vi "ContactsDC.vi"() -> ()   [LabVIEW 2017]
uses:
  <vilib>/Utility/file.llb/Write To Spreadsheet File (DBL).vi
panel:
  in  "Test first # contacts (#<16)":i8=15
  out "Resistance":dbl
  out "Array":bool[][](array[boolean])
  in  "GPIB Address":string="12"
  out "String":string
  in  "Start testing the contacts":bool
  out "Output Current (A)":dbl
  out "Output Voltage (V)":dbl
  out "Compliance limit (V)":dbl
  out "Current Range":u16(ring) items=["100 nA", "1 uA", "10 uA", "100 uA", "1 mA", "10 mA", "100 mA", "1 A"]
  out "Voltage Range":u16(ring) items=["200 mV", "2 V", "20 V", "200 V"]
  out "Current (sourse)":dbl
  out "Voltage (sourse)":dbl
  out "ComplianceIndicator":bool
  out "Compliance limit (A)":dbl
  out "Source Function":u16(ring)=1 items=["Current Source", "Voltage Source"]
  out "Sence Mode":u16(ring) items=["2-wire", "4-wire"]
  in  "ON/OFF channel":bool
  out "ON/OFF indicator":bool
  in  "error in (no error)":errorcluster
  out "error out":errorcluster
  # "Channel\nB"
  # "Before start testing contacts make sure that voltage 1 mV is set on channel B,\nchannel is ON, and compliance is 1 uA (1E-6 A) or smaller."
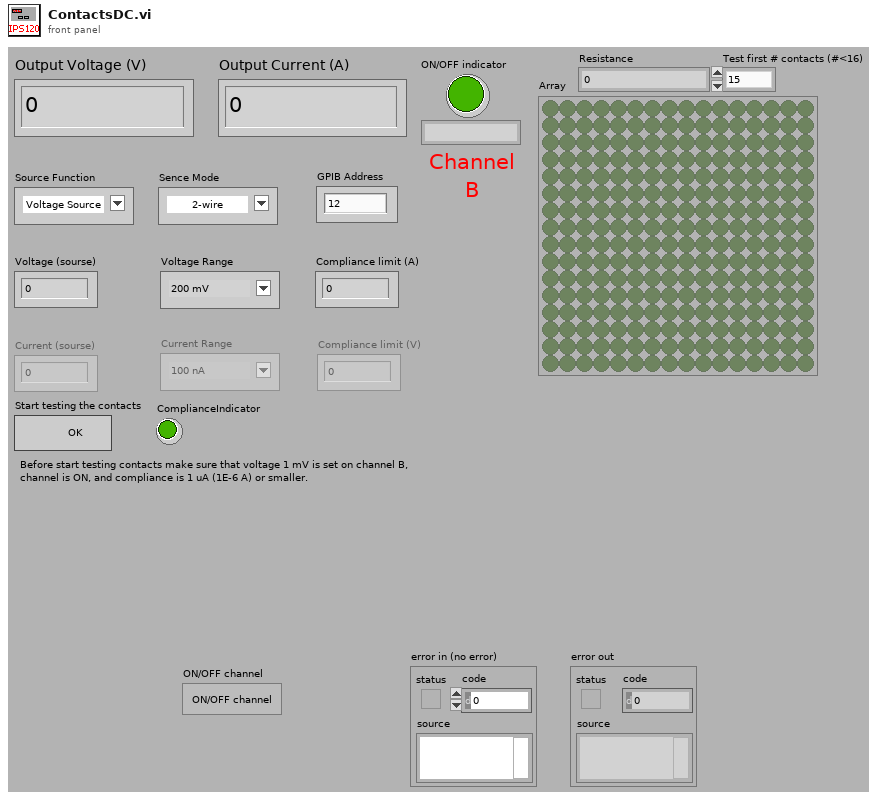
[diagram p1: front panel]
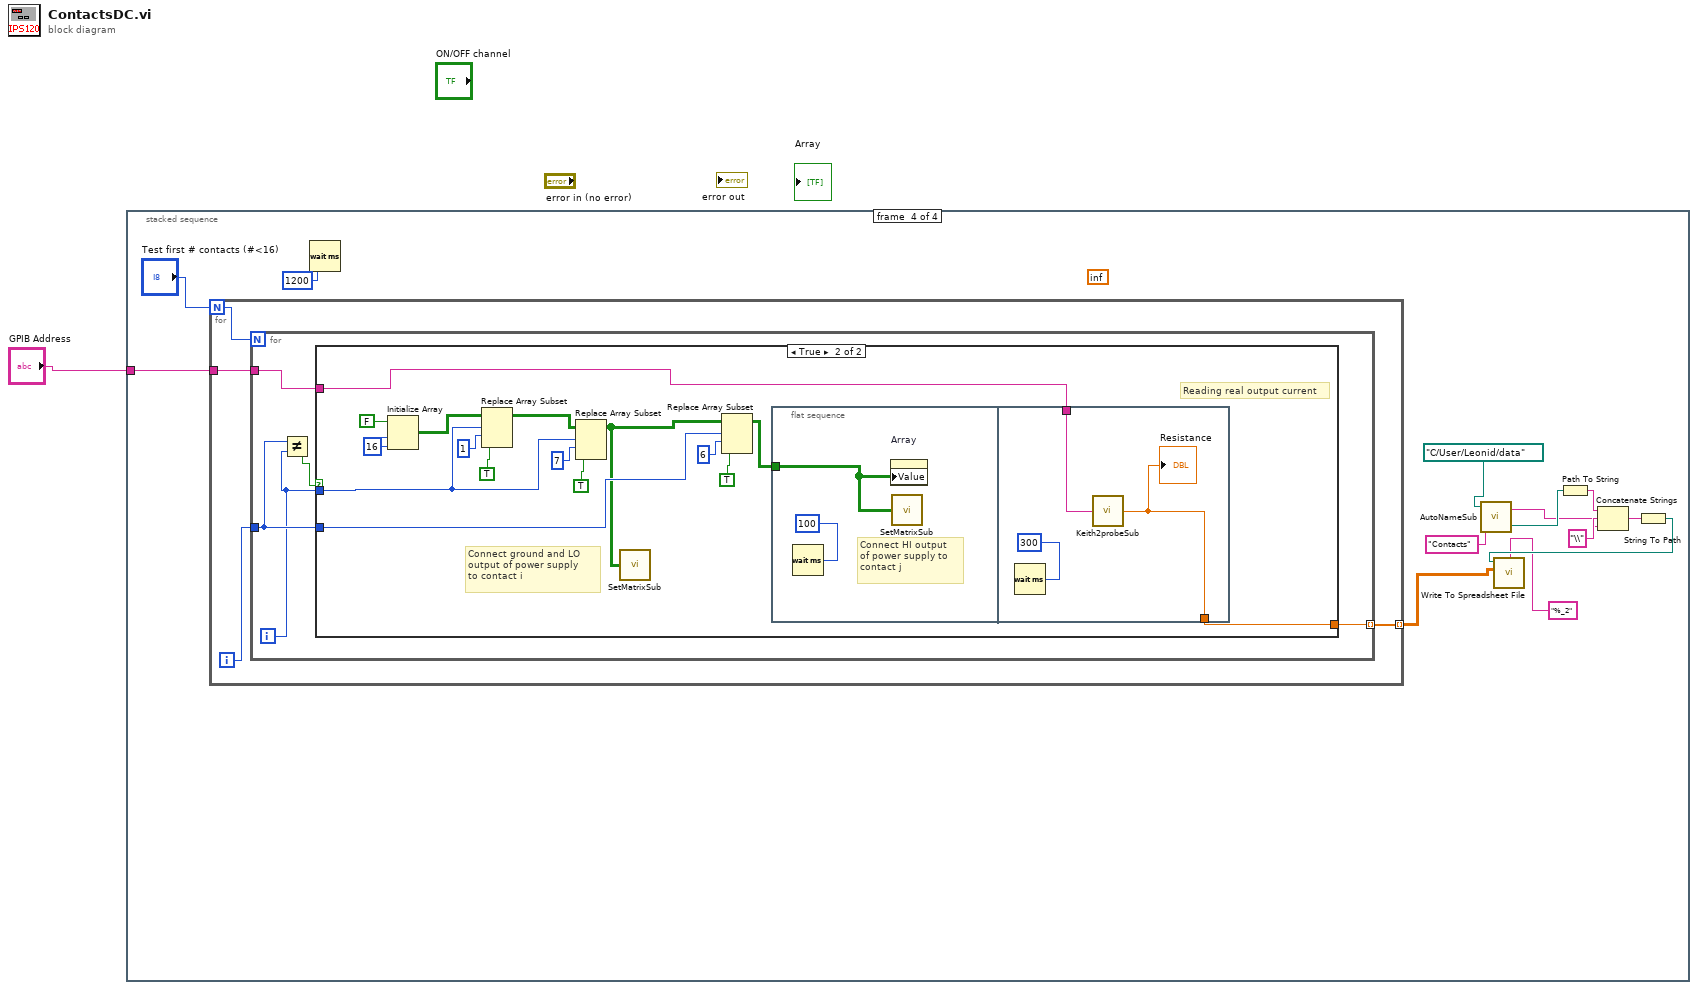
[diagram p0: block diagram]
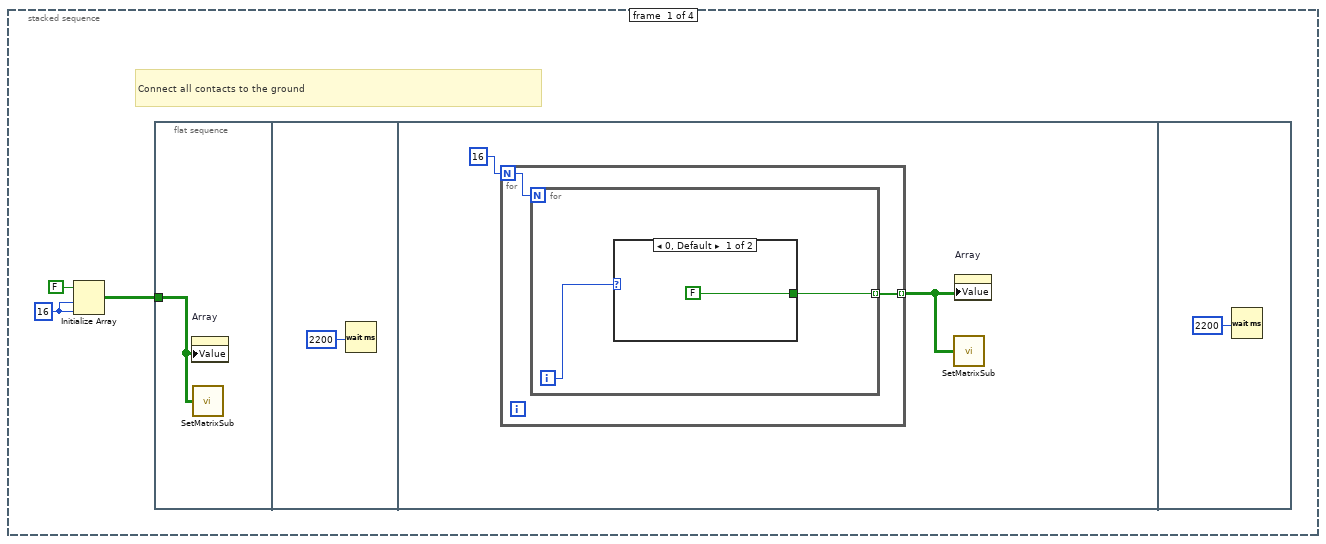
[diagram p2: hidden frame]
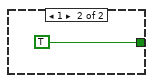
[diagram p3: hidden frame]
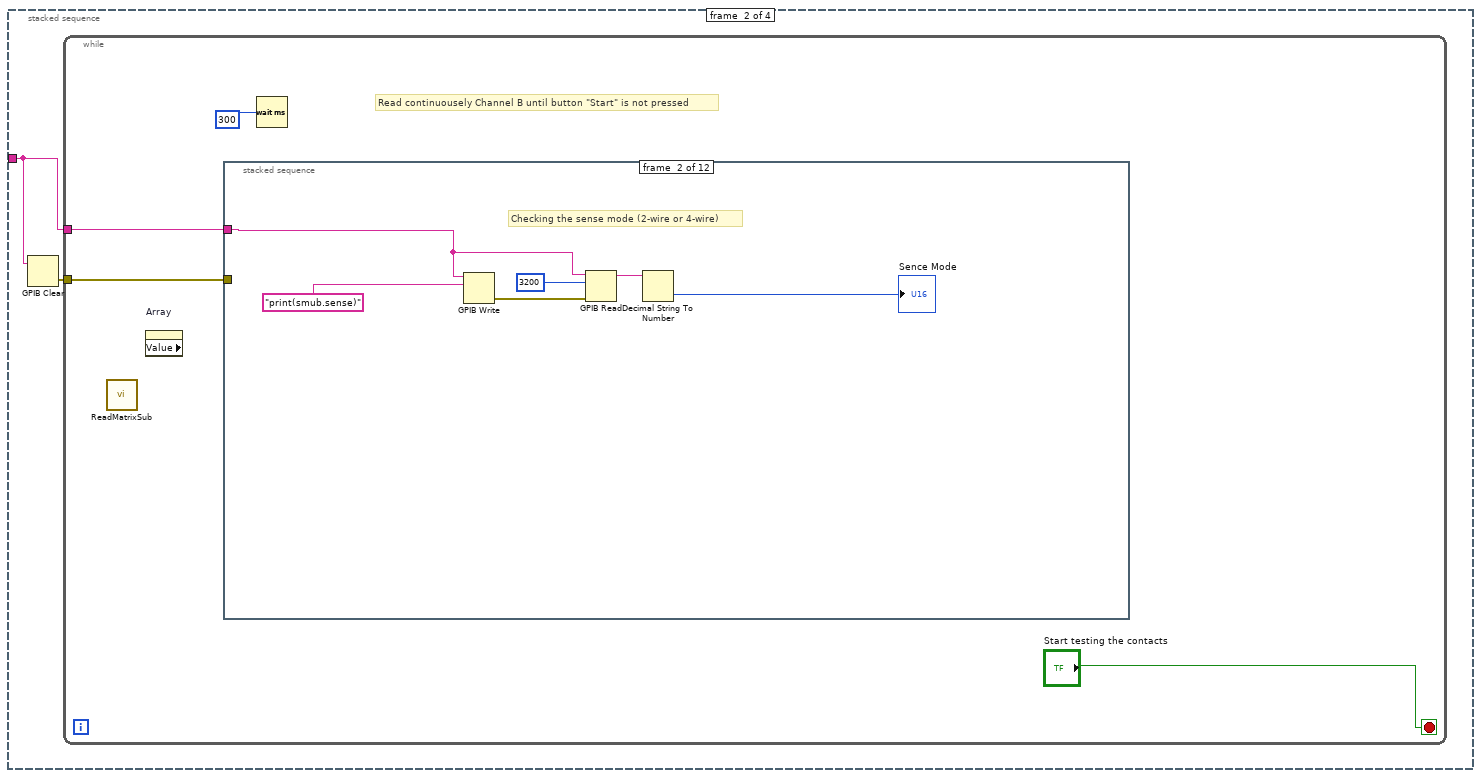
[diagram p4: hidden frame]
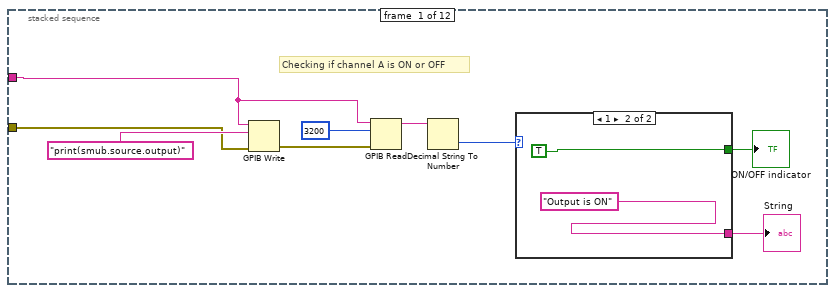
[diagram p5: hidden frame]
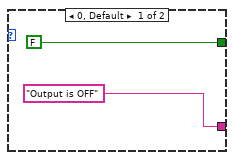
[diagram p6: hidden frame]
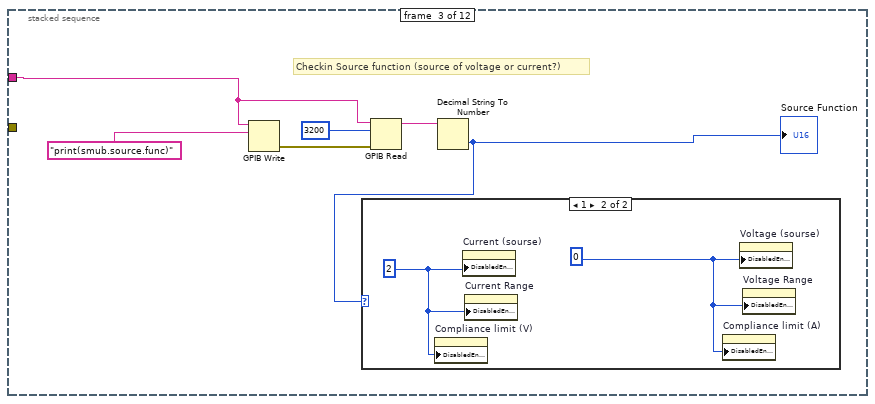
[diagram p7: hidden frame]
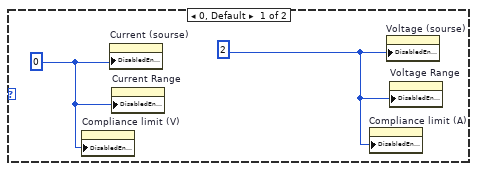
[diagram p8: hidden frame]
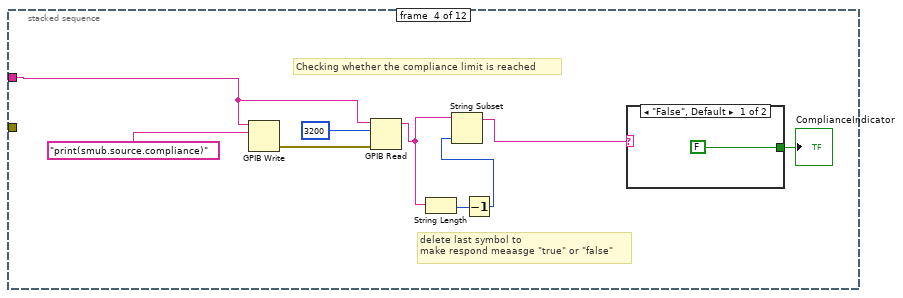
[diagram p9: hidden frame]
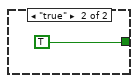
[diagram p10: hidden frame]
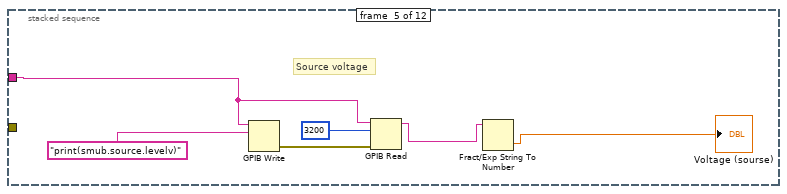
[diagram p11: hidden frame]
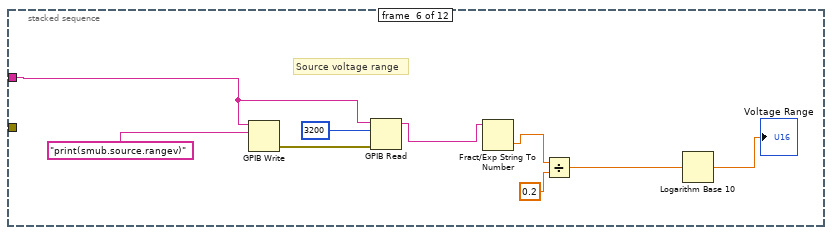
[diagram p12: hidden frame]
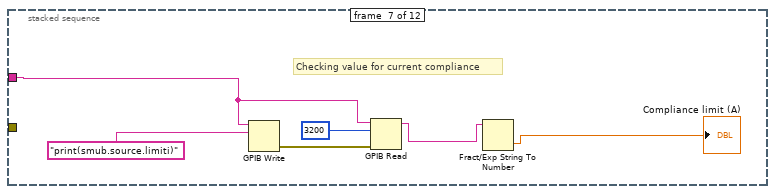
[diagram p13: hidden frame]
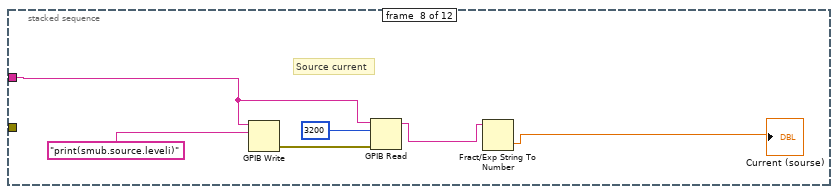
[diagram p14: hidden frame]
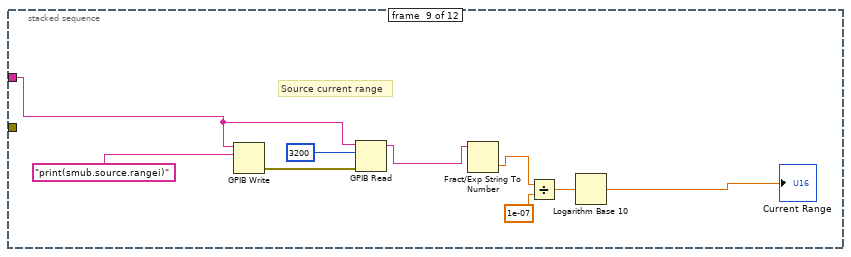
[diagram p15: hidden frame]
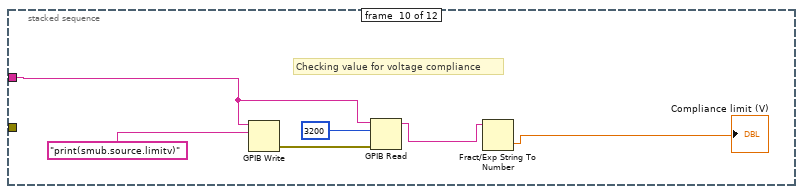
[diagram p16: hidden frame]
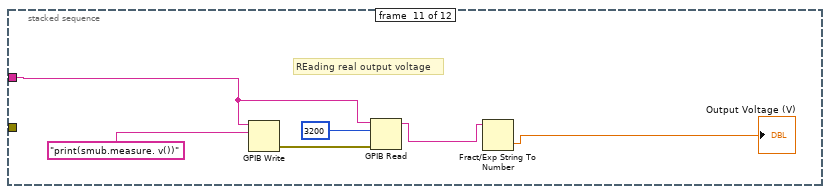
[diagram p17: hidden frame]
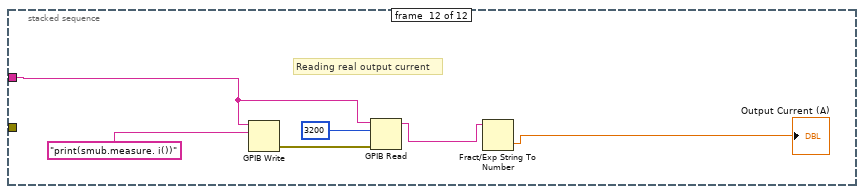
[diagram p18: hidden frame]
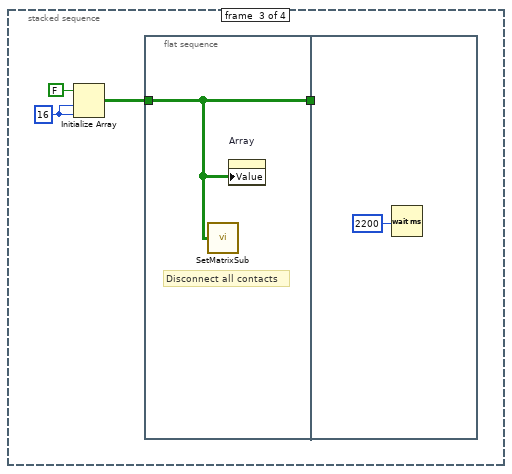
[diagram p19: hidden frame]
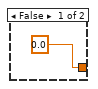
[diagram p20: hidden frame]
diagram:
  n1 = stacked-sequence {
    tunnel: "GPIB Address" -> [_ w17 _ w134]
    frame #0 {
      w3 = 16
      # "Connect all contacts to the ground"
      n2 = Initialize Array(FALSE, w3, w3) -> (w2:bool[][])
      n3 = flat-sequence {
        tunnel: w2 -> [w5]
        frame #0 {
          n4 = property on="Array" class="Arr (strict)"("Value"=w5) -> ()  [unwired: 2 in, 2 out]
          n5 = call "SetMatrixSub.vi"("Array"=w5) -> ()  [unwired: 1 in]
        }
        frame #1 {
          n6 = Wait (ms)(milliseconds to wait=2200) -> ()  [unwired: 1 out]
        }
        frame #2 {
          n7 = for {
            N: 16 -> [w9]
            tunnel: [w10] -> w7 mode=indexing
            n8 = for {
              N: w9 -> [_]
              tunnel: [w12] -> w10 mode=indexing
              i -> [w11]
              n9 = case shown="0, Default" w11 {
                tunnel: [FALSE TRUE] -> w12
                frame 0, Default {
                }
                frame 1 {
                }
              }
            }
          }
          n10 = call "SetMatrixSub.vi"("Array"=w7) -> ()  [unwired: 1 in]
          n11 = property on="Array" class="Arr (strict)"("Value"=w7) -> ()  [unwired: 2 in, 2 out]
        }
        frame #3 {
          n12 = Wait (ms)(milliseconds to wait=2200) -> ()  [unwired: 1 out]
        }
      }
    }
    frame #1 {
      n13 = GPIB Clear(3:w17) -> (0:w16:errorcluster)  [unwired: 1 in, 1 out]
      n14 = while {
        tunnel: w17 -> [w20]
        tunnel: w16 -> [w18]
        stop <- "Start testing the contacts" stop-if-true
        # "Read continuousely Channel B until button \"Start\" is not pressed"
        n15 = call "ReadMatrixSub.vi"() -> ()  [unwired: 9 in, 3 out]
        n16 = property on="Array" class="Arr (strict)" props=["Value"]() -> ()  [unwired: 2 in, 3 out]
        n17 = stacked-sequence {
          tunnel: w20 -> [w23 w35 w41 w51 w62 w68 w77 w83 w89 w98 w104 w110]
          tunnel: w18 -> [w22 _ _ _ _ _ _ _ _ _ _ _]
          frame #0 {
            # "Checking if channel A is ON or OFF"
            n18 = GPIB Write(0:w23, 1:"print(smub.source.output)", 3:w22) -> (6:w30:errorcluster)  [unwired: 2 in, 1 out]
            n19 = GPIB Read(0:w23, 1:3200, 3:w30) -> (5:w27:string)  [unwired: 2 in, 2 out]
            n20 = Decimal String To Number(string=w27) -> (number=w26:i32)  [unwired: 2 in, 1 out]
            n21 = case shown="1" w26 {
              tunnel: [FALSE TRUE] -> w25
              tunnel: ["Output is OFF" "Output is ON"] -> w24
              frame 0, Default {
              }
              frame 1 {
              }
            }
            "ON/OFF indicator" <- w25
            "String" <- w24
          }
          frame #1 {
            # "Checking the sense mode (2-wire or 4-wire)"
            n22 = GPIB Write(0:w35, 1:"print(smub.sense)") -> (6:w40:errorcluster)  [unwired: 3 in, 1 out]
            n23 = GPIB Read(0:w35, 1:3200, 3:w40) -> (5:w37:string)  [unwired: 2 in, 2 out]
            n24 = Decimal String To Number(string=w37) -> (number=→"Sence Mode":i32)  [unwired: 2 in, 1 out]
          }
          frame #2 {
            # "Checkin Source function (source of voltage or current?)"
            n25 = GPIB Write(0:w41, 1:"print(smub.source.func)") -> (6:w46:errorcluster)  [unwired: 3 in, 1 out]
            n26 = GPIB Read(0:w41, 1:3200, 3:w46) -> (5:w43:string)  [unwired: 2 in, 2 out]
            n27 = Decimal String To Number(string=w43) -> (number=w42:i32)  [unwired: 2 in, 1 out]
            "Source Function" <- w42
            n28 = case shown="1" w42 {
              frame 0, Default {
                w47 = 2
                w48 = 0
                n29 = property on="Compliance limit (V)" class="DigNum (strict)"("DisabledEnum"=w48) -> ()  [unwired: 2 in, 2 out]
                n30 = property on="Current (sourse)" class="DigNum (strict)"("DisabledEnum"=w48) -> ()  [unwired: 2 in, 2 out]
                n31 = property on="Current Range" class="Ring (strict)"("DisabledEnum"=w48) -> ()  [unwired: 2 in, 2 out]
                n32 = property on="Compliance limit (A)" class="DigNum (strict)"("DisabledEnum"=w47) -> ()  [unwired: 2 in, 2 out]
                n33 = property on="Voltage (sourse)" class="DigNum (strict)"("DisabledEnum"=w47) -> ()  [unwired: 2 in, 2 out]
                n34 = property on="Voltage Range" class="Ring (strict)"("DisabledEnum"=w47) -> ()  [unwired: 2 in, 2 out]
              }
              frame 1 {
                w49 = 0
                w50 = 2
                n35 = property on="Compliance limit (V)" class="DigNum (strict)"("DisabledEnum"=w50) -> ()  [unwired: 2 in, 2 out]
                n36 = property on="Current (sourse)" class="DigNum (strict)"("DisabledEnum"=w50) -> ()  [unwired: 2 in, 2 out]
                n37 = property on="Current Range" class="Ring (strict)"("DisabledEnum"=w50) -> ()  [unwired: 2 in, 2 out]
                n38 = property on="Compliance limit (A)" class="DigNum (strict)"("DisabledEnum"=w49) -> ()  [unwired: 2 in, 2 out]
                n39 = property on="Voltage (sourse)" class="DigNum (strict)"("DisabledEnum"=w49) -> ()  [unwired: 2 in, 2 out]
                n40 = property on="Voltage Range" class="Ring (strict)"("DisabledEnum"=w49) -> ()  [unwired: 2 in, 2 out]
              }
            }
          }
          frame #3 {
            # "delete last symbol to\nmake respond meaasge \"true\" or \"false\""
            # "Checking whether the compliance limit is reached"
            n41 = GPIB Write(0:w51, 1:"print(smub.source.compliance)") -> (6:w59:errorcluster)  [unwired: 3 in, 1 out]
            n42 = GPIB Read(0:w51, 1:3200, 3:w59) -> (5:w53:string)  [unwired: 2 in, 2 out]
            n43 = String Length(string=w53) -> (length=w55:i32)
            n44 = Decrement(x=w55) -> (x-1=w54:i32)
            n45 = String Subset(string=w53, length (rest)=w54) -> (substring=w52:string)  [unwired: 1 in]
            n46 = case shown="\"False\", Default" w52 {
              tunnel: [FALSE TRUE] -> w56
              frame "False", Default {
              }
              frame "true" {
              }
            }
            "ComplianceIndicator" <- w56
          }
          frame #4 {
            # "Source voltage"
            n47 = GPIB Write(0:w62, 1:"print(smub.source.levelv)") -> (6:w67:errorcluster)  [unwired: 3 in, 1 out]
            n48 = GPIB Read(0:w62, 1:3200, 3:w67) -> (5:w64:string)  [unwired: 2 in, 2 out]
            n49 = Fract/Exp String To Number(string=w64) -> (number=→"Voltage (sourse)":dbl)  [unwired: 3 in, 1 out]
          }
          frame #5 {
            # "Source voltage range"
            n50 = GPIB Write(0:w68, 1:"print(smub.source.rangev)") -> (6:w76:errorcluster)  [unwired: 3 in, 1 out]
            n51 = GPIB Read(0:w68, 1:3200, 3:w76) -> (5:w73:string)  [unwired: 2 in, 2 out]
            n52 = Fract/Exp String To Number(string=w73) -> (number=w71:dbl)  [unwired: 3 in, 1 out]
            n53 = Divide(x=w71, y=0.2) -> (x/y=w70:dbl)
            n54 = Logarithm Base 10(1:w70) -> (0:→"Voltage Range":dbl)
          }
          frame #6 {
            # "Checking value for current compliance"
            n55 = GPIB Write(0:w77, 1:"print(smub.source.limiti)") -> (6:w82:errorcluster)  [unwired: 3 in, 1 out]
            n56 = GPIB Read(0:w77, 1:3200, 3:w82) -> (5:w79:string)  [unwired: 2 in, 2 out]
            n57 = Fract/Exp String To Number(string=w79) -> (number=→"Compliance limit (A)":dbl)  [unwired: 3 in, 1 out]
          }
          frame #7 {
            # "Source current"
            n58 = GPIB Write(0:w83, 1:"print(smub.source.leveli)") -> (6:w88:errorcluster)  [unwired: 3 in, 1 out]
            n59 = GPIB Read(0:w83, 1:3200, 3:w88) -> (5:w85:string)  [unwired: 2 in, 2 out]
            n60 = Fract/Exp String To Number(string=w85) -> (number=→"Current (sourse)":dbl)  [unwired: 3 in, 1 out]
          }
          frame #8 {
            # "Source current range"
            n61 = GPIB Write(0:w89, 1:"print(smub.source.rangei)") -> (6:w97:errorcluster)  [unwired: 3 in, 1 out]
            n62 = GPIB Read(0:w89, 1:3200, 3:w97) -> (5:w94:string)  [unwired: 2 in, 2 out]
            n63 = Fract/Exp String To Number(string=w94) -> (number=w92:dbl)  [unwired: 3 in, 1 out]
            n64 = Divide(x=w92, y=1e-07) -> (x/y=w91:dbl)
            n65 = Logarithm Base 10(1:w91) -> (0:→"Current Range":dbl)
          }
          frame #9 {
            # "Checking value for voltage compliance"
            n66 = GPIB Write(0:w98, 1:"print(smub.source.limitv)") -> (6:w103:errorcluster)  [unwired: 3 in, 1 out]
            n67 = GPIB Read(0:w98, 1:3200, 3:w103) -> (5:w100:string)  [unwired: 2 in, 2 out]
            n68 = Fract/Exp String To Number(string=w100) -> (number=→"Compliance limit (V)":dbl)  [unwired: 3 in, 1 out]
          }
          frame #10 {
            # "REading real output voltage"
            n69 = GPIB Write(0:w104, 1:"print(smub.measure. v())") -> (6:w109:errorcluster)  [unwired: 3 in, 1 out]
            n70 = GPIB Read(0:w104, 1:3200, 3:w109) -> (5:w106:string)  [unwired: 2 in, 2 out]
            n71 = Fract/Exp String To Number(string=w106) -> (number=→"Output Voltage (V)":dbl)  [unwired: 3 in, 1 out]
          }
          frame #11 {
            # "Reading real output current"
            n72 = GPIB Write(0:w110, 1:"print(smub.measure. i())") -> (6:w115:errorcluster)  [unwired: 3 in, 1 out]
            n73 = GPIB Read(0:w110, 1:3200, 3:w115) -> (5:w112:string)  [unwired: 2 in, 2 out]
            n74 = Fract/Exp String To Number(string=w112) -> (number=→"Output Current (A)":dbl)  [unwired: 3 in, 1 out]
          }
        }
        n75 = Wait (ms)(milliseconds to wait=300) -> ()  [unwired: 1 out]
      }
    }
    frame #2 {
      w118 = 16
      n76 = Initialize Array(FALSE, w118, w118) -> (w117:bool[][])
      n77 = flat-sequence {
        tunnel: w117 -> [w120]
        tunnel: [w120] -> w116
        tunnel: w116 -> [_]
        frame #0 {
          # "Disconnect all contacts"
          n78 = call "SetMatrixSub.vi"("Array"=w120) -> ()  [unwired: 1 in]
          n79 = property on="Array" class="Arr (strict)"("Value"=w120) -> ()  [unwired: 2 in, 2 out]
        }
        frame #1 {
          n80 = Wait (ms)(milliseconds to wait=2200) -> ()  [unwired: 1 out]
        }
      }
    }
    frame #3 {
      (unwired) inf
      n81 = for {
        N: "Test first # contacts (#<16)" -> [w137]
        tunnel: w134 -> [w136]
        tunnel: [w135] -> w125 mode=indexing
        i -> [w138]
        n82 = for {
          N: w137 -> [_]
          tunnel: w138 -> [w140]
          tunnel: w136 -> [w143]
          tunnel: [w142] -> w135 mode=indexing
          i -> [w139]
          n83 = Not Equal?(x=w140, y=w139) -> (x != y?=w141:bool)
          n84 = case shown="True" w141 {
            tunnel: w139 -> [_ w146]
            tunnel: w143 -> [_ w160]
            tunnel: [0.0 w159] -> w142
            tunnel: w140 -> [_ w151]
            frame False {
            }
            frame True {
              w157 = 16
              # "Connect ground and LO \noutput of power supply\nto contact i"
              # "Reading real output current"
              n85 = Initialize Array(FALSE, w157, w157) -> (w147:bool[][])
              n86 = Replace Array Subset(array=w147, new element=TRUE, index (row)=w146, index (col)=1) -> (w148:bool[][])
              n87 = Replace Array Subset(array=w148, new element=TRUE, index (row)=w146, index (col)=7) -> (w145:bool[][])
              n88 = call "SetMatrixSub.vi"("Array"=w145) -> ()  [unwired: 1 in]
              n89 = Replace Array Subset(array=w145, new element=TRUE, index (row)=w151, index (col)=6) -> (w152:bool[][])
              n90 = flat-sequence {
                tunnel: w152 -> [w161]
                tunnel: [w164] -> w159
                tunnel: w160 -> [w165]
                frame #0 {
                  # "Connect HI output \nof power supply to \ncontact j"
                  n91 = Wait (ms)(milliseconds to wait=100) -> ()  [unwired: 1 out]
                  n92 = property on="Array" class="Arr (strict)"("Value"=w161) -> ()  [unwired: 2 in, 2 out]
                  n93 = call "SetMatrixSub.vi"("Array"=w161) -> ()  [unwired: 1 in]
                }
                frame #1 {
                  n94 = Wait (ms)(milliseconds to wait=300) -> ()  [unwired: 1 out]
                  n95 = call "Keith2probeSub.vi"("GPIB Address"=w165) -> ("Numeric"=w164:dbl)
                  "Resistance" <- w164
                }
              }
            }
          }
        }
      }
      n96 = Wait (ms)(milliseconds to wait=1200) -> ()  [unwired: 1 out]
      n97 = call "AutoNameSub.vi"("Custom Folder"="Contacts", "User Data Folder"=path "C:/User/Leonid/data") -> ("created path"=w130:path, "String"=w129:string)  [unwired: 2 in]
      n98 = Path To String(path=w130) -> (string=w131:string)
      n99 = Concatenate Strings(w131, "\\", w129) -> (w133:string)
      n100 = String To Path(string=w133) -> (path=w128:path)
      n101 = call-poly <vilib>:"Write To Spreadsheet File.vi"("format (%.3f)"="%_2", "2D data"=w125, "file path (dialog if empty)"=w128) -> ()  [unwired: 5 in, 1 out]
    }
  }
